vi "Doc Builder - Replace Spaces with Underscores.vi"(4 "String":string) -> (1 "String out":string)   [LabVIEW 2011]
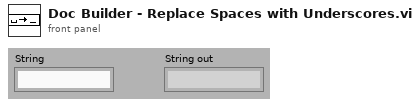
[diagram p1: front panel]
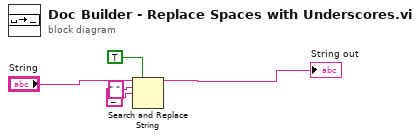
[diagram p0: block diagram]
diagram:
  n1 = Search and Replace String(replace all?=TRUE ("replace all? (F)"), input string="String", search string=" ", replace string="_" ("replace string (\"\")")) -> (result string=→"String out":string)  [unwired: 4 in, 3 out]
